vi "Get_NavXAngle.vi"(8 "error in (no error)":errorcluster, 11 "DriveBase in":refnum<class "DriveBase.lvclass">) -> (0 "error out":errorcluster, 2 "NavX Angle":dbl, 3 "DriveBase out":refnum<class "DriveBase.lvclass">)   [LabVIEW 2016, in "DriveBase.lvclass"]
uses:
  DriveBase.lvclass
  DriveBase.lvclass/DriveBase.ctl
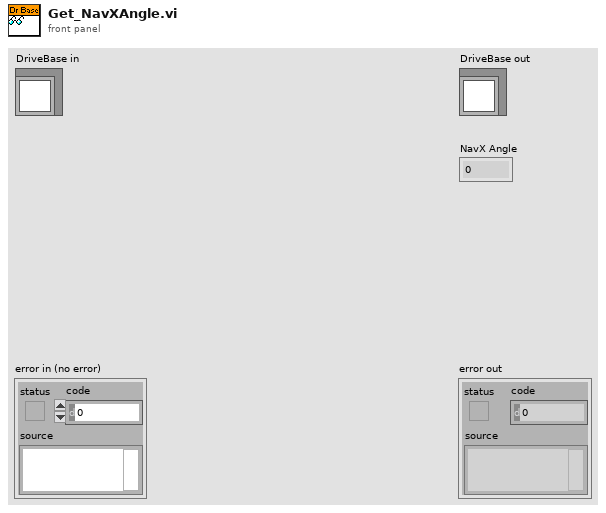
[diagram p1: front panel]
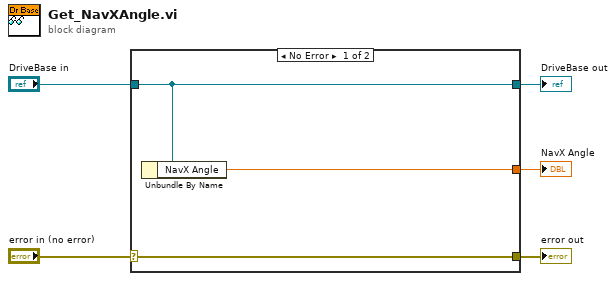
[diagram p0: block diagram]
diagram:
  n1 = case shown="No Error" "error in (no error)" {
    selector: "error in (no error)" -> [w8 w9]
    tunnel: [w8 w9] -> w4
    tunnel: [w7 w10] -> w2
    tunnel: "DriveBase in" -> [w7 w10]
    tunnel: [w6 _] -> w1
    frame No Error {
      n2 = Unbundle By Name(w7) -> ("NavX Angle"=w6:dbl)
    }
    frame Error {
    }
  }
  "error out" <- w4
  "DriveBase out" <- w2
  "NavX Angle" <- w1
